vi "Pulse Duration change.vi"(8 "error in (no error)":errorcluster, 11 "Pressure Control in":refnum<class "Pressure Control.lvclass">) -> (0 "error out":errorcluster, 3 "Pressure Control out":refnum<class "Pressure Control.lvclass">)   [LabVIEW 2014, in "Pressure Control.lvclass"]
uses:
  Pressure Control/Pressure Control.lvclass
  TTL/TTL.lvclass
  Pressure Control/Pressure Control.lvclass/Pressure Control.ctl
panel:
  in  "TTL.lvclass":refnum<class "TTL.lvclass">
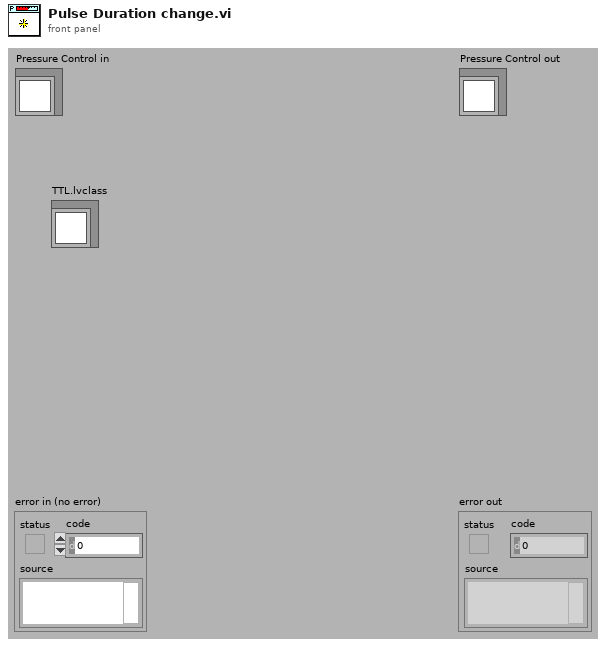
[diagram p1: front panel]
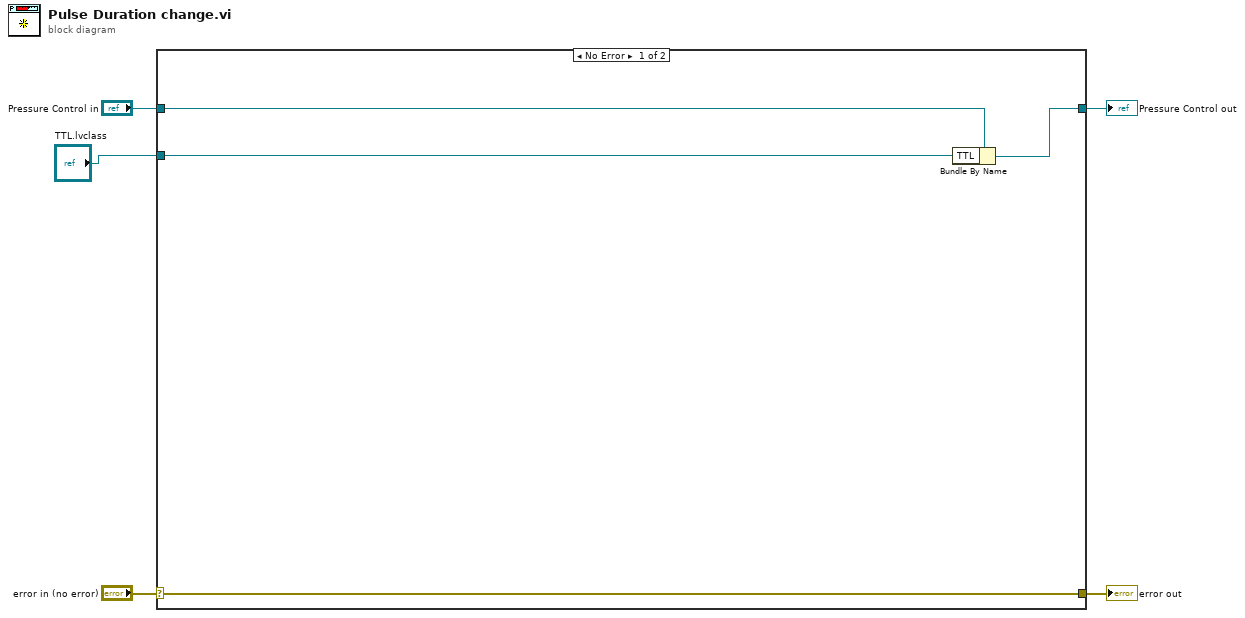
[diagram p0: block diagram]
diagram:
  n1 = case shown="No Error" "error in (no error)" {
    selector: "error in (no error)" -> [w8 w11]
    tunnel: [w8 w11] -> w4
    tunnel: [w9 w10] -> w2
    tunnel: "Pressure Control in" -> [w7 w10]
    tunnel: "TTL.lvclass" -> [w6 _]
    frame No Error {
      n2 = Bundle By Name(cluster=w7, "TTL"=w6) -> (w9:refnum<class "Pressure Control.lvclass">)
    }
    frame Error {
    }
  }
  "error out" <- w4
  "Pressure Control out" <- w2
